vi "Лабораторная №1 Задание 3_2.vi"() -> ()   [LabVIEW 2017]
panel:
  in  "stop":bool
  in  "Knob":dbl(knob) scale=0.0..10.0
  out "Waveform Graph":dynamicdata(graph)
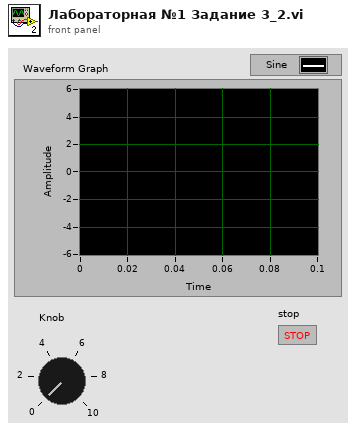
[diagram p1: front panel]
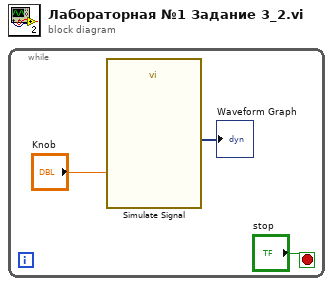
[diagram p0: block diagram]
diagram:
  n1 = while {
    stop <- "stop" stop-if-true
    n2 = call "Simulate Signal"("Amplitude"="Knob") -> ("Sine"=→"Waveform Graph":dynamicdata)  [unwired: 13 in, 1 out]
  }
